vi "TestListFieldSymbols.vi"() -> ()   [LabVIEW 2015, in "SysLog.lvlib"]
uses:
  <vilib>/numeric/LVNumericRepresentation.ctl
  <vilib>/Utility/Data Type/Type Definitions/Unit Info.ctl
  <vilib>/Utility/Data Type/Type Definitions/Unit Type.ctl
  Funktionstasten/Betriebsart.ctl
  Seiten/Erweiterte Konfig/Dichtheitstest Umfang.ctl
  SysLog.lvlib
  <vilib>/Utility/Data Type/NI_Data Type.lvlib
  Funktionstasten/Funktionstasten.lvlib
  Seiten/Erweiterte Konfig/Erweiterte Konfig.lvlib
panel:
  out "Dezimal-Integer-String":string
  out "Representation 2":T1 caption="Darstellung"
  out "Units":T2[](array[typedef]) caption="Einheit"
  out "error out":errorcluster caption="Fehler (Ausgang)"
  out "Enum Names 2":string[](array[string]) caption="Enum-Namen"
  out "Dichtheitstestumfang":string
  out "error in (no error)":errorcluster
  out "Betriebsart":string
  out "Representation":T1 caption="Darstellung"
  out "Enum Names":string[](array[string]) caption="Enum-Namen"
  in  "Boolean":bool=TRUE
  out "resulting string":string
  out "Fehler (Ausgang)":errorcluster
  out "Anzahl der Ersetzungen":i32
  out "Ergebnis-String":string
  out "Array (Ausgang)":string[](array[string])
  in  "filename":string
  in  "Filter":string="SystemLogHistory_cRIO.txt"
  out "Übereinstimmender Teil-String nach Filter":string
  in  "SysLogIcon":enum16{"OK", "Warnung", "Fehler"}(ring)
  in  "Listenfeld":i32(listbox)
  out "Numerisch":i32
  out "Nach Teil-String":string
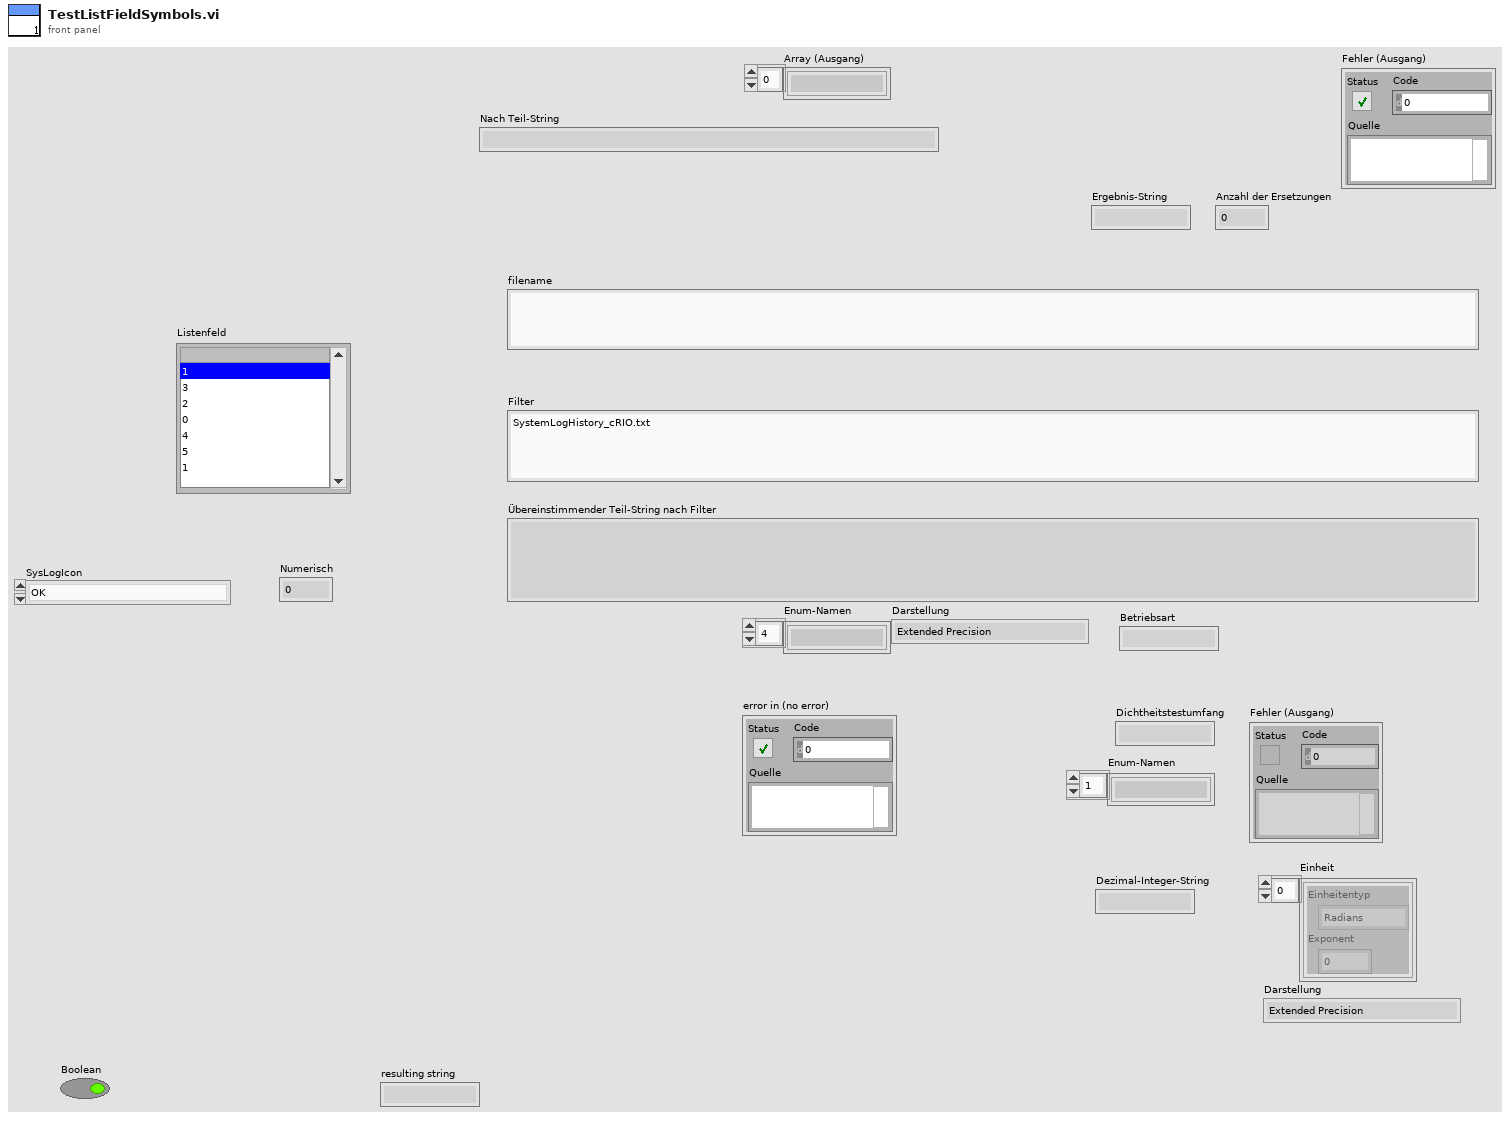
[diagram p1: front panel]
types:
  T1 = typedef "LVNumericRepresentation.ctl" = enum32{"Extended Precision", "Double Precision", "Single Precision", "Long", "Word", "Byte", "Unsigned Long", "Unsigned Word", "Unsigned Byte", "Complex Extended", "Complex Double", "Complex Single", "Quad", "Unsigned Quad", "Fixed-Point"}
  T2 = typedef "NI_Data Type.lvlib/Unit Info.ctl" = cluster{"Unit Type":T3, "Exponent":i16}
  T3 = typedef "NI_Data Type.lvlib/Unit Type.ctl" = enum16{"Radians", "Steradians", "Seconds", "Meters", "Kilograms", "Amperes", "Kelvins", "Moles", "Candelas", "InvalidUnit"}
  T4 = typedef "Erweiterte Konfig.lvlib/Dichtheitstest Umfang.ctl" = u16
  T5 = typedef "Funktionstasten.lvlib/Betriebsart.ctl" = enum16{"Manuell", "Remote", "Bitparallel"}
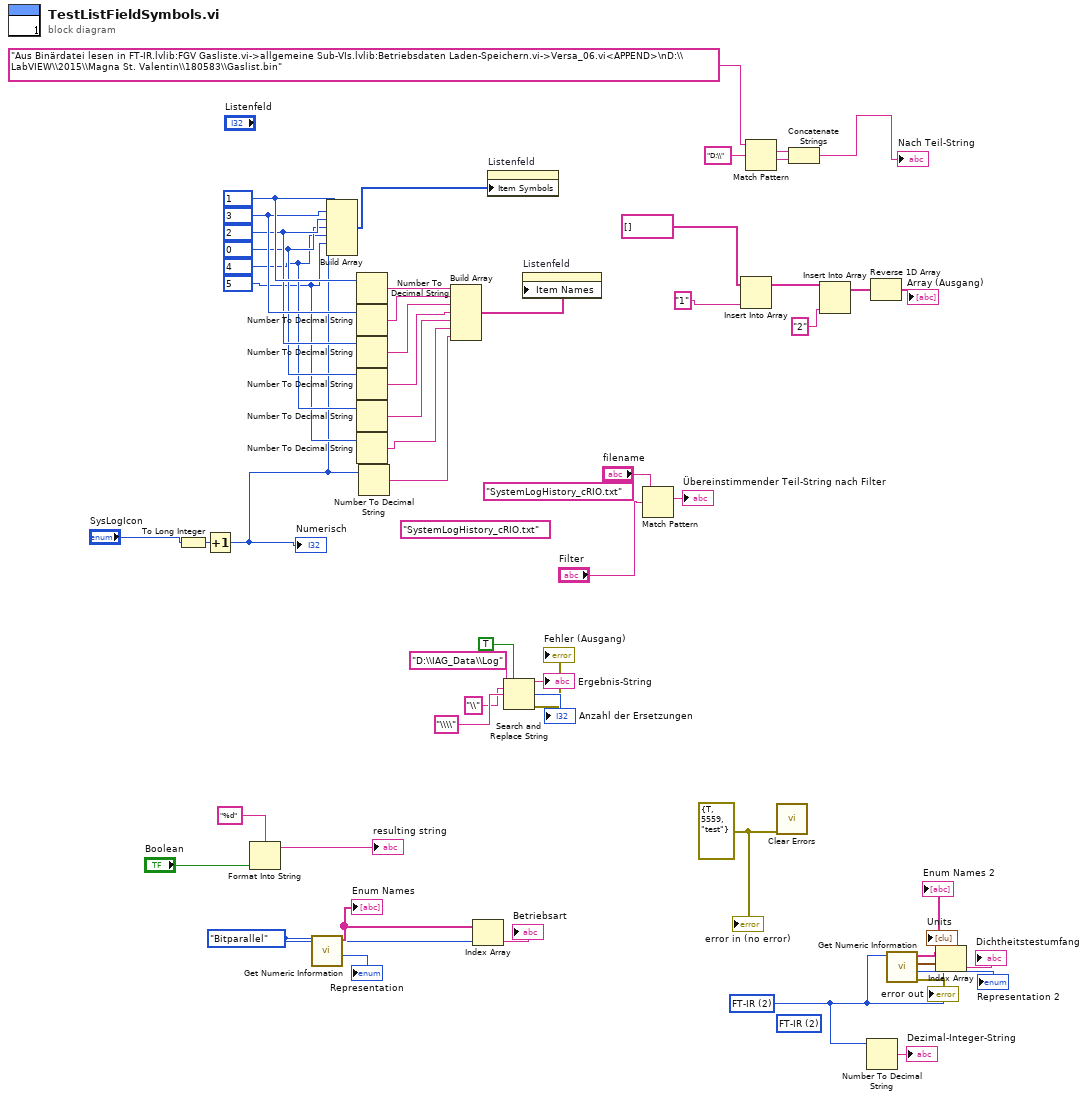
[diagram p0: block diagram]
diagram:
  (unwired) T4 2 items=["Pumpe / Filter / FT-IR", "Filter / FT-IR", "FT-IR"] ("Dichtheitstest Umfang")
  w2 = T4 2 items=["Pumpe / Filter / FT-IR", "Filter / FT-IR", "FT-IR"] ("Dichtheitstest Umfang")
  w8 = errorcluster {"status"=TRUE, "code"=5559, "source"="test"} ("error in (no error)")
  w10 = Betriebsart."Bitparallel" ("Betriebsart")
  (unwired) "SystemLogHistory_cRIO.txt" ("String")
  (unwired) "SystemLogHistory_cRIO.txt" ("String")
  w41 = 5
  w42 = 4
  w43 = 0
  w44 = 2
  w45 = 3
  w48 = 1
  n1 = To Long Integer(number="SysLogIcon") -> (32bit integer=w35:i32)
  n2 = Increment(x=w35) -> (x+1=w32:i32)
  "Numerisch" <- w32
  n3 = Format Into String(format string="%d" ("Format-String"), "Boolean") -> (resulting string=→"resulting string":string)  [unwired: 2 in, 1 out]
  n4 = call <vilib>:"Get Numeric Information.vi"("Variant"=w10) -> ("Representation"=→"Representation":T1, "Enum Names"=w11:string[])  [unwired: 7 in, 2 out]
  "Enum Names" <- w11
  n5 = Build Array(w48, w45, w44, w43, w42, w41, w32) -> (w49:i32[])
  n6 = Number To Decimal String(number=w48) -> (decimal integer string=w47:string)  [unwired: 1 in]
  n7 = Number To Decimal String(number=w45) -> (decimal integer string=w40:string)  [unwired: 1 in]
  n8 = Number To Decimal String(number=w44) -> (decimal integer string=w39:string)  [unwired: 1 in]
  n9 = Number To Decimal String(number=w43) -> (decimal integer string=w38:string)  [unwired: 1 in]
  n10 = Number To Decimal String(number=w42) -> (decimal integer string=w37:string)  [unwired: 1 in]
  n11 = Number To Decimal String(number=w41) -> (decimal integer string=w36:string)  [unwired: 1 in]
  n12 = Number To Decimal String(number=w32) -> (decimal integer string=w33:string)  [unwired: 1 in]
  n13 = Build Array(w47, w40, w39, w38, w37, w36, w33) -> (w46:string[])
  n14 = Index Array(array=w11, index=w10) -> (element=→"Betriebsart":string)
  n15 = property on="Listenfeld" class="Listenfeld (strikt)"("Item Symbols"=w49) -> ()  [unwired: 2 in, 2 out]
  n16 = Search and Replace String(replace all?=TRUE ("Alle ersetzen? (F)"), input string="D:\\IAG_Data\\Log", search string="\\", replace string="\\\\") -> (result string=→"Ergebnis-String":string, number of replacements=→"Anzahl der Ersetzungen":i32, error out=→"Fehler (Ausgang)":errorcluster)  [unwired: 4 in, 1 out]
  n17 = property on="Listenfeld" class="Listenfeld (strikt)"("Item Names"=w46) -> ()  [unwired: 2 in, 2 out]
  n18 = Match Pattern(string="filename", regular expression="Filter") -> (match substring=→"Übereinstimmender Teil-String nach Filter":string)  [unwired: 1 in, 3 out]
  n19 = Insert Into Array(array=string[] [], new element="1") -> (w26:string[])  [unwired: 1 in]
  n20 = Match Pattern(string="Aus Binärdatei lesen in FT-IR.lvlib:FGV Gasliste.vi->allgemeine Sub-VIs.lvlib:Betriebsdaten Laden-Speichern.vi->Versa_06.vi<APPEND>\nD:\\LabVIEW\\2015\\Magna St. Valentin\\180583\\Gaslist.bin" ("source"), regular expression="D:\\") -> (match substring=w52:string, after substring=w51:string)  [unwired: 1 in, 2 out]
  n21 = call <vilib>:"Clear Errors.vi"("error in (no error)"=w8) -> ()  [unwired: 5 in, 2 out]
  n22 = Concatenate Strings(w52, w51) -> (→"Nach Teil-String":string)
  n23 = Insert Into Array(array=w26, new element="2") -> (w24:string[])  [unwired: 1 in]
  n24 = Number To Decimal String(number=w2) -> (decimal integer string=→"Dezimal-Integer-String":string)  [unwired: 1 in]
  n25 = Reverse 1D Array(array=w24) -> (reversed array=→"Array (Ausgang)":string[])
  n26 = call <vilib>:"Get Numeric Information.vi"("Variant"=w2) -> ("error out"=→"error out":errorcluster, "Representation"=→"Representation 2":T1, "Units"=→"Units":T2[], "Enum Names"=w7:string[])  [unwired: 7 in]
  "Enum Names 2" <- w7
  n27 = Index Array(array=w7, index=w2) -> (element=→"Dichtheitstestumfang":string)
  "error in (no error)" <- w8
